vi "Alpha Numeric Sort 1D String Array.vi"(3 "Descending? (F)":bool, 4 "1D String[]":string[](array[string])) -> (0 "Sorted Index[]":i32[](array[numeric]), 1 "Sorted 1D String[]":string[](array[string]))   [LabVIEW 2016, in "SLL String.lvlib"]
doc: "Alpha Numeric Sorting of 1D String Array so that strings are ordered like File 1, File 2..File 10 instead of the usual sorting like File 1, File 10, File 2.."
uses:
  SLL String.lvlib
  _Typedefs/Sortable Alpha Numeric Cluster.ctl
  <vilib>/regexp/Match Regular Expression.xnode
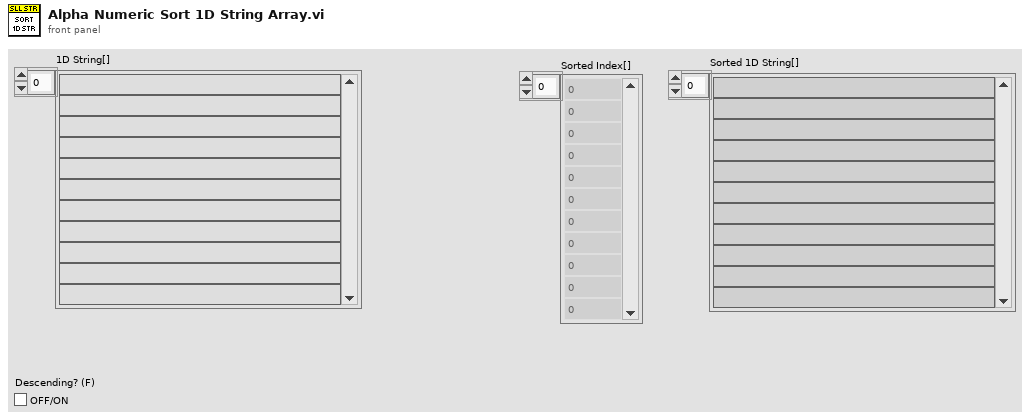
[diagram p1: front panel]
types:
  T1 = typedef "SLL String.lvlib/Sortable Alpha Numeric Cluster.ctl" = cluster{"Numeric[]":dbl[], "String":string}
  T2 = cluster{"Sortable Cluster[]":T1[], "Input String":string, "Index":i32}
  T3 = cluster{"Sortable Cluster[]":T1[], "Input String":string, "Index":i32}[]
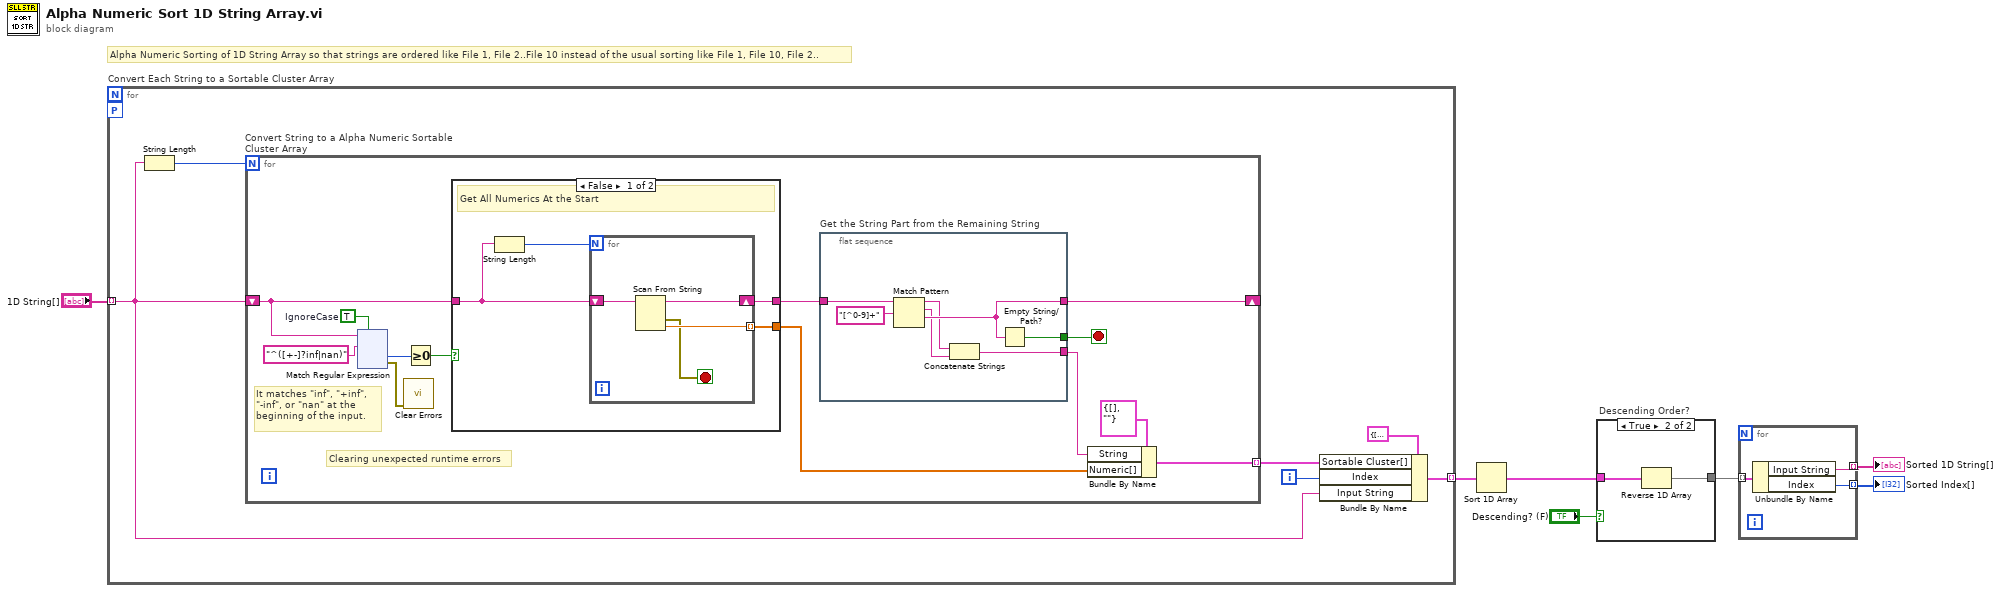
[diagram p0: block diagram]
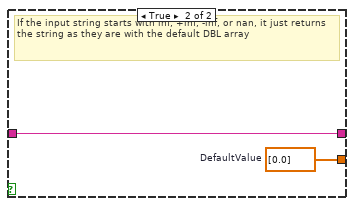
[diagram p3: hidden frame]
diagram:
  # "Alpha Numeric Sorting of 1D String Array so that strings are ordered like File 1, File 2..File 10 instead of the usual sorting like File 1, File 10, File 2.."
  n1 = for "Convert Each String to a Sortable Cluster Array" {
    tunnel: "1D String[]" -> [w8] mode=indexing
    workers-P: _ -> [_]
    tunnel: [w9] -> w6 mode=indexing
    i -> [w10]
    n2 = String Length(string=w8) -> (length=w13:i32)
    n3 = for "Convert String to a Alpha Numeric Sortable Cluster Array" {
      N: w13 -> [_]
      shift-right: [w22] -> _
      shift-left: w8 -> [w20]
      tunnel: [w23] -> w11 mode=indexing
      stop <- w21 stop-if-true
      w19 = TRUE  # IgnoreCase
      # "Clearing unexpected runtime errors"
      # "It matches \"inf\", \"+inf\", \n\"-inf\", or \"nan\" at the \nbeginning of the input."
      n4 = xnode "Match Regular Expression"("input string"=w20, "regular expression"="^([+-]?inf|nan)", "ignore case? (F)"=w19) -> ("offset past match"=w17:i32, "error out"=w15:errorcluster)  [unwired: 3 in, 3 out]
      n5 = call <vilib>:"Clear Errors.vi"("error in (no error)"=w15) -> ()  [unwired: 5 in, 2 out]
      n6 = Greater Or Equal To 0?(x=w17) -> (x >= 0?=w16:bool)
      n7 = case shown="False" w16 {
        tunnel: [w147 w153] -> w26
        tunnel: [w146 w152] -> w24
        tunnel: w20 -> [w145 w153]
        frame False {
          # "Get All Numerics At the Start"
          n8 = String Length(string=w145) -> (length=w144:i32)
          n9 = for "Get All Numerics At the Start" {
            N: w144 -> [_]
            shift-right: [w150] -> w147
            shift-left: w145 -> [w151]
            tunnel: [w149] -> w146 mode=indexing
            stop <- w148 stop-if-true
            n10 = Scan From String(input string=w151) -> (remaining string=w150:string, error out=w148:errorcluster, output 1=w149:dbl)  [unwired: 4 in, 1 out]
          }
        }
        frame True {
          w152 = dbl[] [0.0]  # DefaultValue
          # "If the input string starts with inf, +inf, -inf, or nan, it just returns the string as they are with the default DBL array"
        }
      }
      n11 = flat-sequence "Get the String Part from the Remaining String" {
        tunnel: w26 -> [w159]
        tunnel: [w157] -> w22
        tunnel: [w160] -> w21
        tunnel: [w154] -> w14
        frame #0 {
          n12 = Match Pattern(string=w159, regular expression="[^0-9]+" ("format string")) -> (before substring=w156:string, match substring=w155:string, after substring=w157:string)  [unwired: 1 in, 1 out]
          n13 = Concatenate Strings(w156, w155) -> (w154:string)
          n14 = Empty String/Path?(string/path=w157) -> (empty?=w160:bool)
        }
      }
      n15 = Bundle By Name(cluster=T1 {"Numeric[]"=[], "String"=""}, "String"=w14, "Numeric[]"=w24) -> (w23:T1)
    }
    n16 = Bundle By Name(cluster=T2 {"Sortable Cluster[]"=[], "Input String"="", "Index"=0}, "Sortable Cluster[]"=w11, "Index"=w10, "Input String"=w8) -> (w9:T2)
  }
  n17 = Sort 1D Array(array=w6) -> (sorted array=w5:T3)
  n18 = case "Descending Order?" shown="True" "Descending? (F)" {
    tunnel: w5 -> [w161 w163]
    tunnel: [w161 w162] -> w2
    frame False {
    }
    frame True {
      n19 = Reverse 1D Array(array=w163) -> (reversed array=w162:T3)
    }
  }
  n20 = for {
    tunnel: w2 -> [w166] mode=indexing
    tunnel: [w165] -> w4 mode=indexing
    tunnel: [w164] -> w3 mode=indexing
    n21 = Unbundle By Name(w166) -> ("Input String"=w165:string, "Index"=w164:i32)
  }
  "Sorted 1D String[]" <- w4
  "Sorted Index[]" <- w3
